vi "Set Multipliers (timed).vi"(0 "timeout (ms)":i32=5000, 7 "new mult":dbl, 11 "error in (no error)":errorcluster) -> (15 "error out":errorcluster={"status"=FALSE, "code"=0, "source"="."})   [LabVIEW 2015]
uses:
  PXI Globals.vi
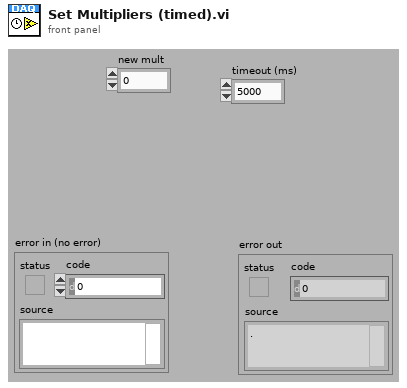
[diagram p1: front panel]
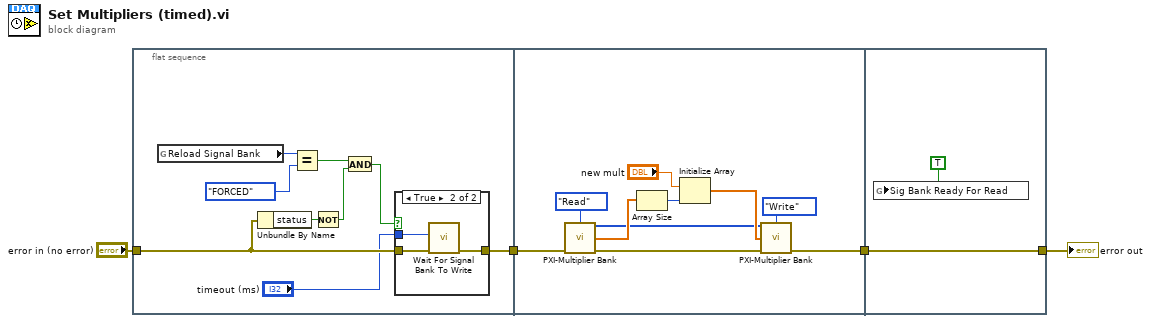
[diagram p0: block diagram]
diagram:
  n1 = flat-sequence {
    tunnel: "error in (no error)" -> [w6]
    tunnel: [w13] -> w3
    tunnel: w3 -> [w23]
    tunnel: [w21] -> w2
    tunnel: [w28] -> w1
    tunnel: w2 -> [w28]
    frame #0 {
      n2 = global read "PXI Globals.vi" "Reload Signal Bank"() -> (w8:enum32{"OFF", "ENABLED", "FORCED"})
      n3 = Unbundle By Name(w6) -> ("status"=w10:bool)
      n4 = Equal?(x=w8, y=enum16{"OFF", "ENABLED", "FORCED"}."FORCED") -> (x = y?=w12:bool)
      n5 = Not(x=w10) -> (.not. x?=w11:bool)
      n6 = And(x=w12, y=w11) -> (x .and. y?=w7:bool)
      n7 = case shown="True" w7 {
        tunnel: w6 -> [w14 w17]
        tunnel: [w14 w16] -> w13
        tunnel: "timeout (ms)" -> [_ w15]
        frame False {
        }
        frame True {
          n8 = call "Wait For Signal Bank To Write.vi"("error in (no error)"=w17, "timeout (ms)"=w15) -> ("error out"=w16:errorcluster)  [unwired: 8 in, 1 out]
        }
      }
    }
    frame #1 {
      n9 = call "PXI-Multiplier Bank.vi"("Action"=enum16{"Init", "Write", "Read"}."Read", "error in (no error)"=w23) -> ("Channels"=w19:i32[], "Multipliers out"=w24:dbl[], "error out"=w22:errorcluster)  [unwired: 11 in]
      n10 = Array Size(array=w24) -> (size(s)=w27:i32)
      n11 = Initialize Array("new mult", w27) -> (w20:dbl[])
      n12 = call "PXI-Multiplier Bank.vi"("AO Channels"=w19, "Action"=enum16{"Init", "Write", "Read"}."Write", "Multipliers"=w20, "error in (no error)"=w22) -> ("error out"=w21:errorcluster)  [unwired: 9 in, 2 out]
    }
    frame #2 {
      n13 = global write "PXI Globals.vi" "Sig Bank Ready For Read"(TRUE) -> ()
    }
  }
  "error out" <- w1
